vi "Find Custom Device.vi"(8 "error in":errorcluster, 10 "name":string, 11 "target in":refnum<k24>) -> (0 "error out":errorcluster, 2 "custom device":u64, 3 "target out":refnum<k24>)   [LabVIEW 2020, in "AIM ARINC 664 Scripting.lvlib"]
doc: "Within the specified target, this VI searches for all the AIM ARINC 664 custom devices and returns references to found <b>custom devices</b>."
uses:
  AIM ARINC 664 Scripting.lvlib
  NationalInstruments.VeriStand.SystemDefinitionAPI
  Constants.vi
panel:
  in  "error message":string="The item with the specified name is not an instance of this custom device."
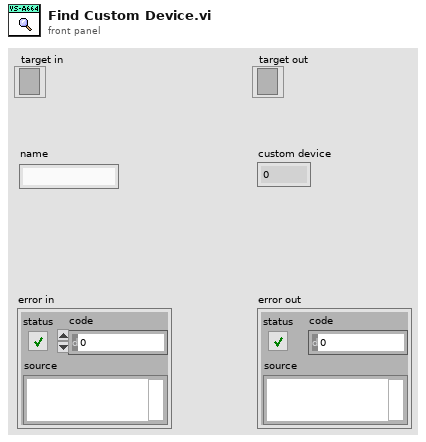
[diagram p1: front panel]
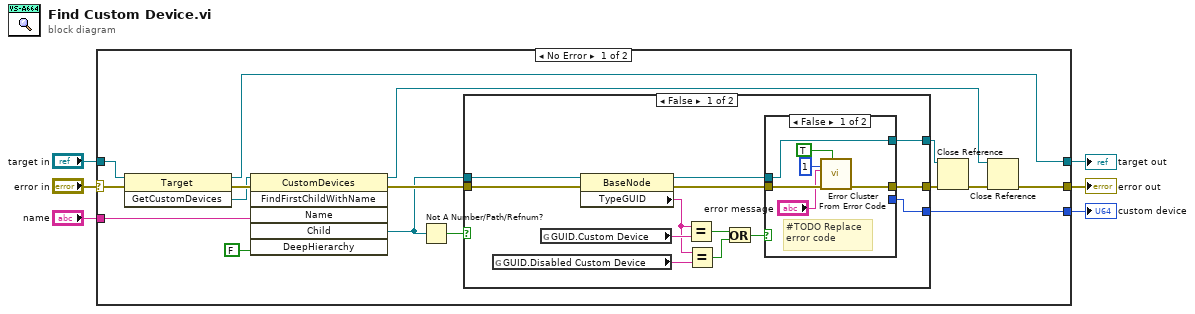
[diagram p0: block diagram]
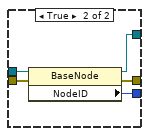
[diagram p2: hidden frame]
diagram:
  n1 = case shown="No Error" "error in" {
    selector: "error in" -> [w17 w50]
    tunnel: "target in" -> [w18 w49]
    tunnel: [w12 w50] -> w4
    tunnel: [w9 _] -> w1
    tunnel: [w14 w49] -> w3
    tunnel: "name" -> [w11 _]
    frame No Error {
      n2 = invoke on="Invoke Node" class="Target" method="GetCustomDevices"(reference=w18, error in=w17) -> (reference out=w14:refnum<k24>, error out=w22:errorcluster, "GetCustomDevices"=w21:refnum<k24>)  [unwired: 1 in]
      n3 = invoke on="Invoke Node" class="CustomDevices" method="FindFirstChildWithName"(reference=w21, error in=w22, "Name"=w11, "DeepHierarchy"=FALSE) -> (reference out=w15:refnum<k24>, error out=w13:errorcluster, "Child"=w10:refnum<k24>)  [unwired: 2 in, 3 out]
      n4 = Not A Number/Path/Refnum?(number/path/refnum=w10) -> (NaN/Path/Refnum?=w8:bool)
      n5 = case shown="False" w8 {
        tunnel: [w35 w47] -> w20
        tunnel: [w34 w48] -> w19
        tunnel: w13 -> [w32 w48]
        tunnel: w10 -> [w31 w47]
        tunnel: [w33 _] -> w9
        frame False {
          n6 = global read "Constants.vi" "GUID.Disabled Custom Device"() -> (w27:string)
          n7 = global read "Constants.vi" "GUID.Custom Device"() -> (w30:string)
          n8 = property on="Property Node" class="BaseNode"(reference=w31, error in=w32) -> (reference out=w28:refnum<k24>, error out=w29:errorcluster, "TypeGUID"=w26:string)
          n9 = Equal?(x=w26, y=w30) -> (x = y?=w24:bool)
          n10 = Equal?(x=w26, y=w27) -> (x = y?=w25:bool)
          n11 = Or(x=w24, y=w25) -> (x .or. y?=w23:bool)
          n12 = case shown="False" w23 {
            tunnel: [w37 w43] -> w34
            tunnel: w29 -> [w40 w45]
            tunnel: w28 -> [w41 w46]
            tunnel: [w41 w44] -> w35
            tunnel: [_ w42] -> w33
            frame False {
              # "#TODO Replace\nerror code"
              n13 = call <vilib>:"Error Cluster From Error Code.vi"("show call chain? (False)"=TRUE, "error in (no error)"=w40, "error message (\"\")"="error message", "error code (0)"=1) -> ("error out"=w37:errorcluster)  [unwired: 5 in]
            }
            frame True {
              n14 = property on="Property Node" class="BaseNode"(reference=w46, error in=w45) -> (reference out=w44:refnum<k24>, error out=w43:errorcluster, "NodeID"=w42:u64)
            }
          }
        }
        frame True {
        }
      }
      n15 = Close Reference(reference=w20, error in (no error)=w19) -> (error out=w16:errorcluster)
      n16 = Close Reference(reference=w15, error in (no error)=w16) -> (error out=w12:errorcluster)
    }
    frame Error {
    }
  }
  "error out" <- w4
  "target out" <- w3
  "custom device" <- w1
